vi "Updated Editable Nodes.vi"(7 "Channel UI Controls":T1, 11 "Editable Nodes":T2(array[cluster])) -> (3 "Updated Editable Nodes":T2(array[cluster]))   [LabVIEW 2025]
uses:
  Types/Channel UI Controls.ctl
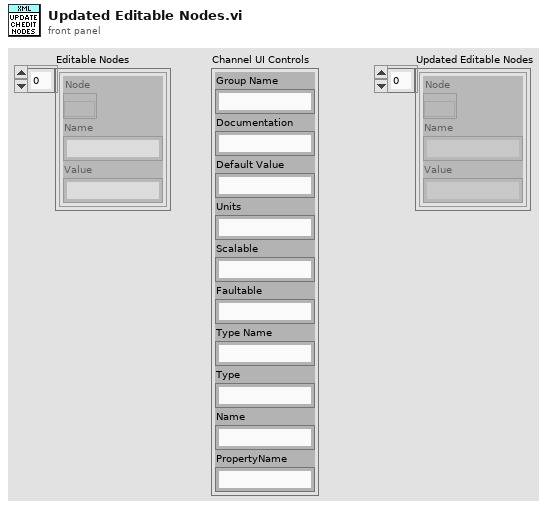
[diagram p1: front panel]
types:
  T1 = typedef "Channel UI Controls.ctl" = cluster{"Group Name":string, "Documentation":string, "Default Value":string, "Units":string, "Scalable":string, "Faultable":string, "Type Name":string, "Type ":string, "Name":string, "PropertyName":string}
  T2 = cluster{"Node":refnum<k20>, "Name":string, "Value":string}[]
  T3 = cluster{"Node":refnum<k20>, "Name":string, "Value":string}
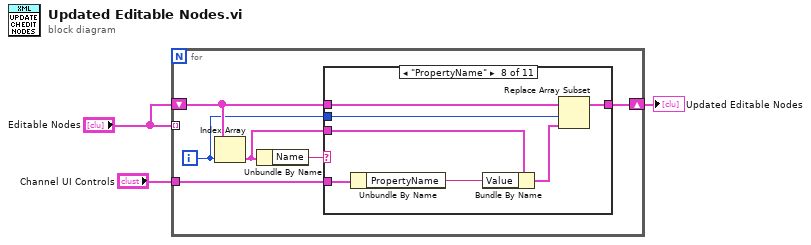
[diagram p0: block diagram]
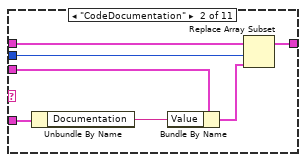
[diagram p3: hidden frame]
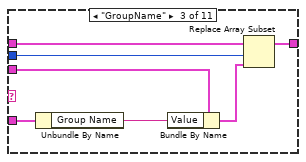
[diagram p4: hidden frame]
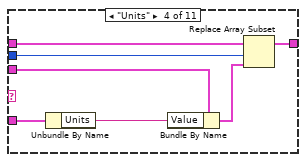
[diagram p5: hidden frame]
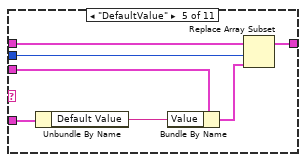
[diagram p6: hidden frame]
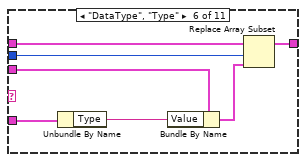
[diagram p7: hidden frame]
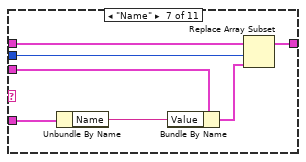
[diagram p8: hidden frame]
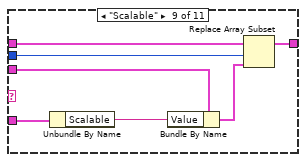
[diagram p9: hidden frame]
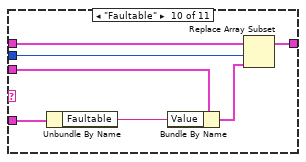
[diagram p10: hidden frame]
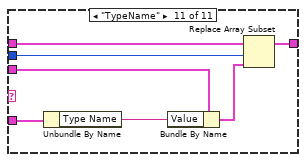
[diagram p11: hidden frame]
diagram:
  n1 = for {
    tunnel: "Editable Nodes" -> [_] mode=indexing
    shift-right: [w5] -> w2
    shift-left: "Editable Nodes" -> [w7]
    tunnel: "Channel UI Controls" -> [w4]
    i -> [w6]
    n2 = Index Array(array=w7, index=w6) -> (element=w8:T3)
    n3 = Unbundle By Name(w8) -> ("Name"=w9:string)
    n4 = case shown="\"PropertyName\"" w9 {
      tunnel: w8 -> [_ w17 w24 w31 w38 w45 w52 w59 w66 w73 w80]
      tunnel: w7 -> [w10 w16 w23 w30 w37 w44 w51 w58 w65 w72 w79]
      tunnel: w6 -> [_ w15 w22 w29 w36 w43 w50 w57 w64 w71 w78]
      tunnel: [w10 w14 w21 w28 w35 w42 w49 w56 w63 w70 w77] -> w5
      tunnel: w4 -> [_ w12 w19 w26 w33 w40 w47 w54 w61 w68 w75]
      frame Default {
      }
      frame "CodeDocumentation" {
        n5 = Unbundle By Name(w12) -> ("Documentation"=w11:string)
        n6 = Bundle By Name(cluster=w17, "Value"=w11) -> (w13:T3)
        n7 = Replace Array Subset(array=w16, new element=w13, index=w15) -> (w14:T2)
      }
      frame "GroupName" {
        n8 = Unbundle By Name(w19) -> ("Group Name"=w18:string)
        n9 = Bundle By Name(cluster=w24, "Value"=w18) -> (w20:T3)
        n10 = Replace Array Subset(array=w23, new element=w20, index=w22) -> (w21:T2)
      }
      frame "Units" {
        n11 = Unbundle By Name(w26) -> ("Units"=w25:string)
        n12 = Bundle By Name(cluster=w31, "Value"=w25) -> (w27:T3)
        n13 = Replace Array Subset(array=w30, new element=w27, index=w29) -> (w28:T2)
      }
      frame "DefaultValue" {
        n14 = Unbundle By Name(w33) -> ("Default Value"=w32:string)
        n15 = Bundle By Name(cluster=w38, "Value"=w32) -> (w34:T3)
        n16 = Replace Array Subset(array=w37, new element=w34, index=w36) -> (w35:T2)
      }
      frame "DataType", "Type" {
        n17 = Unbundle By Name(w40) -> ("Type"=w39:string)
        n18 = Bundle By Name(cluster=w45, "Value"=w39) -> (w41:T3)
        n19 = Replace Array Subset(array=w44, new element=w41, index=w43) -> (w42:T2)
      }
      frame "Name" {
        n20 = Unbundle By Name(w47) -> ("Name"=w46:string)
        n21 = Bundle By Name(cluster=w52, "Value"=w46) -> (w48:T3)
        n22 = Replace Array Subset(array=w51, new element=w48, index=w50) -> (w49:T2)
      }
      frame "PropertyName" {
        n23 = Unbundle By Name(w54) -> ("PropertyName"=w53:string)
        n24 = Bundle By Name(cluster=w59, "Value"=w53) -> (w55:T3)
        n25 = Replace Array Subset(array=w58, new element=w55, index=w57) -> (w56:T2)
      }
      frame "Scalable" {
        n26 = Unbundle By Name(w61) -> ("Scalable"=w60:string)
        n27 = Bundle By Name(cluster=w66, "Value"=w60) -> (w62:T3)
        n28 = Replace Array Subset(array=w65, new element=w62, index=w64) -> (w63:T2)
      }
      frame "Faultable" {
        n29 = Unbundle By Name(w68) -> ("Faultable"=w67:string)
        n30 = Bundle By Name(cluster=w73, "Value"=w67) -> (w69:T3)
        n31 = Replace Array Subset(array=w72, new element=w69, index=w71) -> (w70:T2)
      }
      frame "TypeName" {
        n32 = Unbundle By Name(w75) -> ("Type Name"=w74:string)
        n33 = Bundle By Name(cluster=w80, "Value"=w74) -> (w76:T3)
        n34 = Replace Array Subset(array=w79, new element=w76, index=w78) -> (w77:T2)
      }
    }
  }
  "Updated Editable Nodes" <- w2
